vi "testWriteSpreadsheet.vi"() -> ()   [LabVIEW 2014]
panel:
  in  "Numeric":dbl
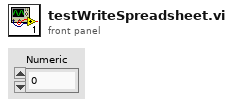
[diagram p1: front panel]
types:
  T1 = enum16{"big-endian, network order", "native, host order", "little-endian"}
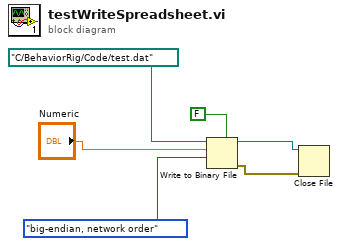
[diagram p0: block diagram]
diagram:
  n1 = Write to Binary File(file (use dialog)=path "C:/BehaviorRig/Code/test.dat", data="Numeric", 5:FALSE ("prepend array or string size? (T)"), 9:T1."big-endian, network order" ("byte order (0:big-endian, network order)")) -> (refnum out=w5:refnum<file>, error out=w4:errorcluster)  [unwired: 2 in, 1 out]
  n2 = Close File(refnum=w5, error in=w4) -> ()  [unwired: 2 out]
